vi "Get stack info.vi"(8 "error in (no error)":errorcluster, 11 "Tomo in":refnum<class "Tomo.lvclass">) -> (0 "error out":errorcluster, 1 "Z start":dbl, 2 "Z stop":dbl, 3 "Tomo out":refnum<class "Tomo.lvclass">, 4 "Y position":dbl, 5 "X position":dbl)   [LabVIEW 2012, in "Tomo.lvclass"]
uses:
  Tomo.lvclass
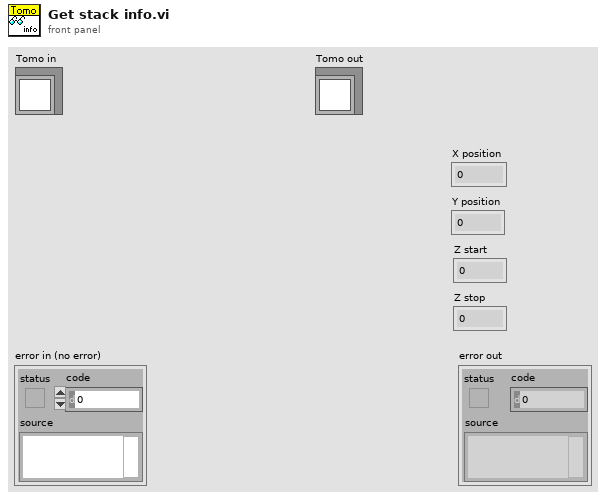
[diagram p1: front panel]
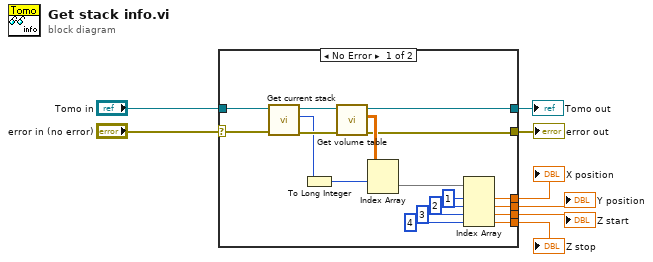
[diagram p0: block diagram]
diagram:
  n1 = case shown="No Error" "error in (no error)" {
    selector: "error in (no error)" -> [w23 w28]
    tunnel: [w14 w28] -> w7
    tunnel: [w13 w27] -> w1
    tunnel: "Tomo in" -> [w26 w27]
    tunnel: [w12 _] -> w6
    tunnel: [w11 _] -> w5
    tunnel: [w10 _] -> w4
    tunnel: [w9 _] -> w3
    frame No Error {
      n2 = call-dynamic "Get current stack.vi"("error in (no error)"=w23, "Tomo in"=w26) -> ("error out"=w24:errorcluster, "Current stack"=w21:u16, "Tomo out"=w25:refnum<class "Tomo.lvclass">)  [unwired: 7 in]
      n3 = To Long Integer(number=w21) -> (32bit integer=w20:i32)
      n4 = call-dynamic "Get volume table.vi"("error in (no error)"=w24, "Tomo in"=w25) -> ("error out"=w14:errorcluster, "Volume table out"=w22:dbl[][], "Tomo out"=w13:refnum<class "Tomo.lvclass">)  [unwired: 7 in]
      n5 = Index Array(array=w22, index (row)=w20) -> (element=w19:dbl[])  [unwired: 1 in]
      n6 = Index Array(array=w19, index #1=1 ("index"), index #2=2 ("index"), index #3=3 ("index"), index #4=4 ("index")) -> (element #1=w12:dbl, element #2=w11:dbl, element #3=w10:dbl, element #4=w9:dbl)
    }
    frame Error {
    }
  }
  "error out" <- w7
  "X position" <- w6
  "Z start" <- w4
  "Y position" <- w5
  "Z stop" <- w3
  "Tomo out" <- w1
